vi "License by time.vi"() -> ()   [LabVIEW 2025]
uses:
  Abstract License/Case.ctl
  <vilib>/Utility/config.llb/Write Key (Double).vi
  <vilib>/Utility/config.llb/Read Key (Double).vi
  <vilib>/Utility/config.llb/NI_LVConfig.lvlib
panel:
  out "String":string
  out "Indicators":bool
  in  "Controls":bool
  out "Time":string
  in  "Install":bool
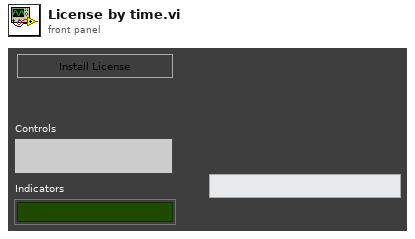
[diagram p1: front panel]
types:
  T1 = typedef "Case.ctl" = enum16{"Init", "idle", "Install", "Get time", "Read file", "Unlicensed", "Licensed", "Check", "Close"}
  T2 = enum8{"Enabled", "Disabled", "Disabled and Grayed Out"}
  T3 = cluster{"Case":T1, "appended path":path, "section":string, "key":string, "TimeReg":dbl, "ActualTime":dbl}
  T4 = typedef "LVDateTimeRec.ctl" = cluster{"fractional second":dbl, "second":i32, "minute":i32, "hour":i32, "day of month":i32, "month":i32, "year":i32, "day of week":i32, "day of year":i32, "DST":i32}
  T5 = typedef "NI_LVConfig.lvlib/Config Data RefNum.ctl" = refnum<k1>
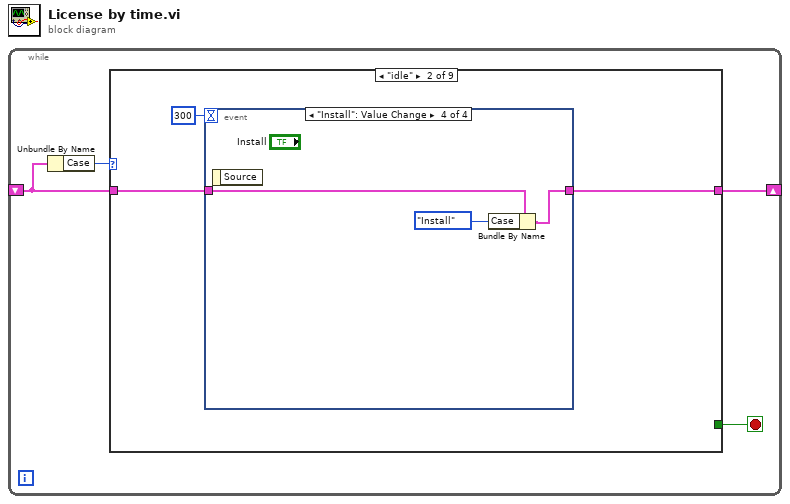
[diagram p0: block diagram]
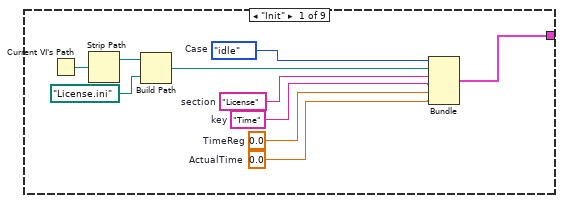
[diagram p2: hidden frame]
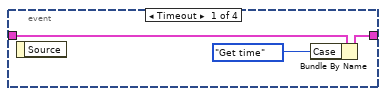
[diagram p3: hidden frame]
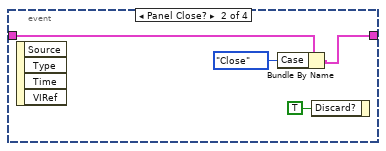
[diagram p4: hidden frame]
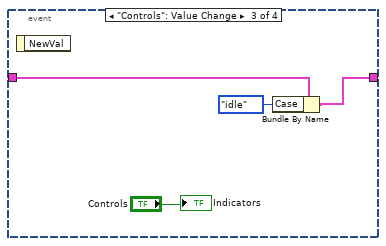
[diagram p5: hidden frame]
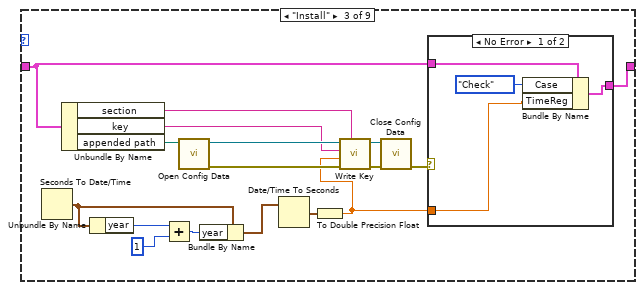
[diagram p6: hidden frame]
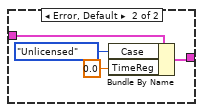
[diagram p7: hidden frame]
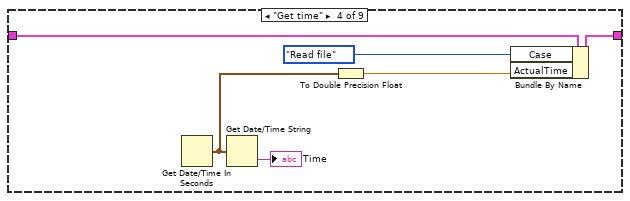
[diagram p8: hidden frame]
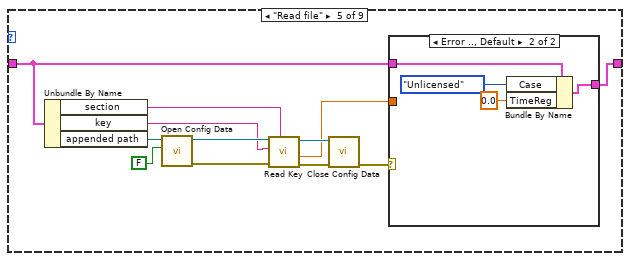
[diagram p9: hidden frame]
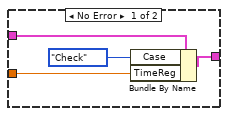
[diagram p10: hidden frame]
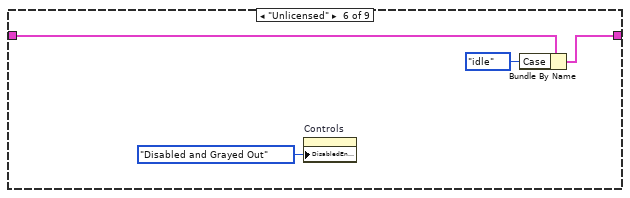
[diagram p11: hidden frame]
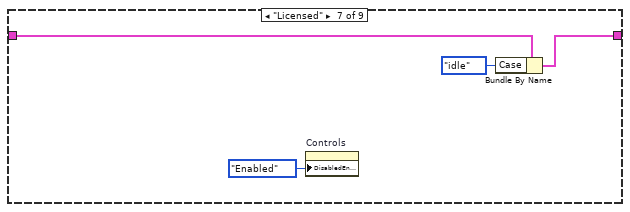
[diagram p12: hidden frame]
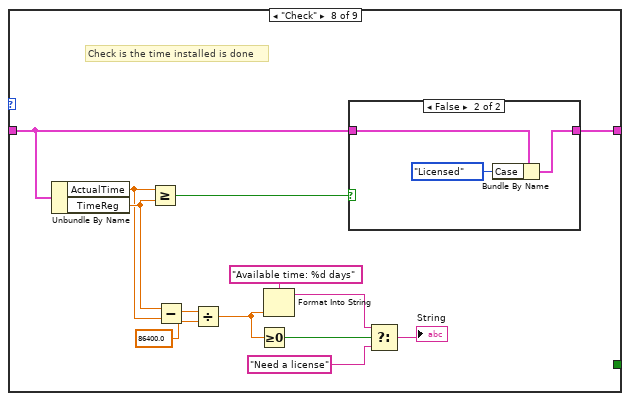
[diagram p13: hidden frame]
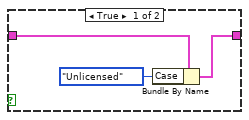
[diagram p14: hidden frame]
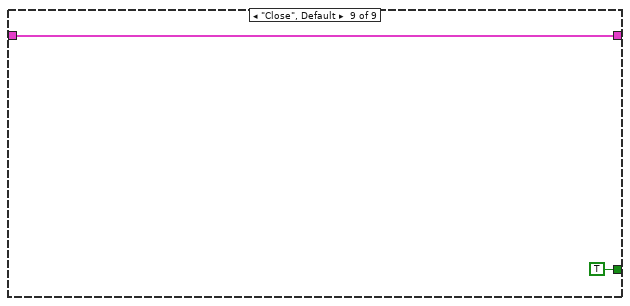
[diagram p15: hidden frame]
diagram:
  n1 = while {
    shift-right: [w1] -> _
    shift-left: _ -> [w3]
    stop <- w4 stop-if-true
    n2 = Unbundle By Name(w3) -> ("Case"=w2:T1)
    n3 = case shown="\"idle\"" w2 {
      tunnel: [_ _ _ _ _ _ _ _ TRUE] -> w4
      tunnel: [w14 w15 w33 w61 w66 w83 w88 w103 w111] -> w1
      tunnel: w3 -> [_ w17 w46 w62 w68 w85 w89 w102 w111]
      frame "Init" {
        w10 = "Time"  # key
        w8 = 0.0  # ActualTime
        w9 = 0.0  # TimeReg
        w12 = "License"  # section
        w11 = Case."idle"  # Case
        n4 = Current VI's Path() -> (path=w13:path)
        n5 = Strip Path(path=w13) -> (stripped path=w7:path)  [unwired: 1 out]
        n6 = Build Path(base path=w7, name or relative path=path "License.ini") -> (appended path=w5:path)
        n7 = Bundle("Case"=w11, "appended path"=w5, "section"=w12, "key"=w10, "TimeReg"=w9, "ActualTime"=w8) -> (w14:T3)  [unwired: 1 in]
      }
      frame "idle" {
        n8 = event shown="[3] \"Install\": Value Change" {
          selector: _ -> [_ _ _ _]
          dyn-events: _ -> [_ _ _ _]
          timeout: 300 -> [_ _ _ _]
          tunnel: [w19 w22 w27 w30] -> w15
          tunnel: w17 -> [w20 w24 w28 w31]
          event Timeout {
            n9 = event-data() -> ()  [unwired: 1 in, 1 out]
            n10 = Bundle By Name(cluster=w20, "Case"=Case."Get time" ("Enum")) -> (w19:T3)
          }
          event Panel Close? {
            n11 = event-data() -> ()  [unwired: 1 in, 4 out]
            n12 = Bundle By Name(cluster=w24, "Case"=Case."Close") -> (w22:T3)
            n13 = event-data("Discard?"=TRUE) -> ()  [unwired: 1 in, 1 out]
          }
          event "Controls": Value Change {
            n14 = event-data() -> ()  [unwired: 1 in, 1 out]
            n15 = Bundle By Name(cluster=w28, "Case"=Case."idle") -> (w27:T3)
            "Indicators" <- "Controls"
          }
          event "Install": Value Change {
            n16 = event-data() -> ()  [unwired: 1 in, 1 out]
            n17 = Bundle By Name(cluster=w31, "Case"=Case."Install" ("Enum")) -> (w30:T3)
          }
        }
      }
      frame "Install" {
        n18 = Seconds To Date/Time() -> (date time rec=w37:T4)  [unwired: 2 in]
        n19 = Unbundle By Name(w46) -> ("section"=w44:string, "key"=w43:string, "appended path"=w48:path)
        n20 = Unbundle By Name(w37) -> ("year"=w36:i32)
        n21 = Add(x=w36, y=1) -> (x+y=w38:i32)
        n22 = call <vilib>:"Open Config Data.vi"("configuration file path"=w48) -> ("error out"=w42:errorcluster, "refnum"=w45:T5)  [unwired: 8 in, 1 out]
        n23 = Bundle By Name(cluster=w37, "year"=w38) -> (w39:T4)
        n24 = Date/Time To Seconds(2:w39) -> (0:w34:timestamp)  [unwired: 1 in]
        n25 = To Double Precision Float(number=w34) -> (double precision float=w32:dbl)
        n26 = call-poly <vilib>:"Write Key.vi"("section"=w44, "error in (no error)"=w42, "value"=w32, "key"=w43, "refnum"=w45) -> ("error out"=w41:errorcluster, "refnum out"=w40:T5)  [unwired: 4 in, 1 out]
        n27 = call <vilib>:"Close Config Data.vi"("error in (no error)"=w41, "refnum"=w40) -> ("error out"=w47:errorcluster)  [unwired: 8 in, 1 out]
        n28 = case shown="No Error" w47 {
          tunnel: w46 -> [w52 w56]
          tunnel: [w51 w55] -> w33
          tunnel: w32 -> [w49 _]
          frame No Error {
            n29 = Bundle By Name(cluster=w52, "Case"=Case."Check", "TimeReg"=w49) -> (w51:T3)
          }
          frame Error, Default {
            n30 = Bundle By Name(cluster=w56, "Case"=Case."Unlicensed", "TimeReg"=0.0) -> (w55:T3)
          }
        }
      }
      frame "Get time" {
        n31 = Get Date/Time In Seconds() -> (seconds since 1Jan1904=w59:timestamp)
        n32 = Get Date/Time String(seconds (now)=w59) -> (time string=→"Time":string)  [unwired: 2 in, 1 out]
        n33 = To Double Precision Float(number=w59) -> (double precision float=w58:dbl)
        n34 = Bundle By Name(cluster=w62, "Case"=Case."Read file", "ActualTime"=w58) -> (w61:T3)
      }
      frame "Read file" {
        n35 = Unbundle By Name(w68) -> ("section"=w64:string, "key"=w63:string, "appended path"=w69:path)
        n36 = call <vilib>:"Open Config Data.vi"("create file if necessary (T)"=FALSE, "configuration file path"=w69) -> ("error out"=w73:errorcluster, "refnum"=w74:T5)  [unwired: 7 in, 1 out]
        n37 = call-poly <vilib>:"Read Key.vi"("section"=w64, "error in (no error)"=w73, "key"=w63, "refnum"=w74) -> ("error out"=w70:errorcluster, "value"=w65:dbl, "refnum out"=w71:T5)  [unwired: 4 in, 1 out]
        n38 = call <vilib>:"Close Config Data.vi"("error in (no error)"=w70, "refnum"=w71) -> ("error out"=w67:errorcluster)  [unwired: 8 in, 1 out]
        n39 = case shown="Error .., Default" w67 {
          tunnel: w68 -> [w78 w82]
          tunnel: [w77 w81] -> w66
          tunnel: w65 -> [w76 _]
          frame No Error {
            n40 = Bundle By Name(cluster=w78, "Case"=Case."Check", "TimeReg"=w76) -> (w77:T3)
          }
          frame Error, Default {
            n41 = Bundle By Name(cluster=w82, "Case"=Case."Unlicensed", "TimeReg"=0.0) -> (w81:T3)
          }
        }
      }
      frame "Unlicensed" {
        n42 = property on="Controls" class="Bool (strict)"("DisabledEnum"=T2."Disabled and Grayed Out" ("Disabled")) -> ()  [unwired: 2 in, 2 out]
        n43 = Bundle By Name(cluster=w85, "Case"=Case."idle") -> (w83:T3)
      }
      frame "Licensed" {
        n44 = property on="Controls" class="Bool (strict)"("DisabledEnum"=T2."Enabled" ("Disabled")) -> ()  [unwired: 2 in, 2 out]
        n45 = Bundle By Name(cluster=w89, "Case"=Case."idle") -> (w88:T3)
      }
      frame "Check" {
        # "Check is the time installed is done"
        n46 = Unbundle By Name(w102) -> ("ActualTime"=w99:dbl, "TimeReg"=w100:dbl)
        n47 = Greater Or Equal?(x=w99, y=w100) -> (x >= y?=w101:bool)
        n48 = Subtract(x=w100, y=w99) -> (x-y=w93:dbl)
        n49 = Divide(x=w93, y=86400.0) -> (x/y=w92:dbl)
        n50 = Greater Or Equal To 0?(x=w92) -> (x >= 0?=w97:bool)
        n51 = Format Into String(format string="Available time: %d days", w92) -> (resulting string=w96:string)  [unwired: 2 in, 1 out]
        n52 = case shown="False" w101 {
          tunnel: w102 -> [w106 w109]
          tunnel: [w105 w108] -> w103
          frame True {
            n53 = Bundle By Name(cluster=w106, "Case"=Case."Unlicensed") -> (w105:T3)
          }
          frame False {
            n54 = Bundle By Name(cluster=w109, "Case"=Case."Licensed") -> (w108:T3)
          }
        }
        n55 = Select(t=w96, s=w97, f="Need a license") -> (s? t:f=→"String":string)
      }
      frame "Close", Default {
      }
    }
  }
